vi "Get Channels From Line.vi"(11 "Line":T1) -> (2 "Channels":refnum<class "TBM channel.lvclass">[](array[class]), 3 "Line 2":T1)   [LabVIEW 2013, in "Modbus Module configuration.lvclass"]
uses:
  Modbus Module configuration.lvclass
  module channel/Modbus Module Channel.lvclass
  Line.ctl
  <vilib>/NI/Tag Bus Module Framework/channel/TBM channel.lvclass
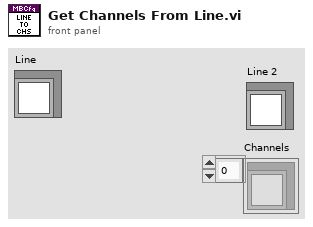
[diagram p1: front panel]
types:
  T1 = typedef "Modbus Module configuration.lvclass/Line.ctl" = refnum<class "Modbus Module Channel.lvclass">
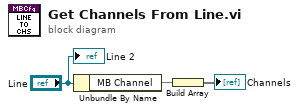
[diagram p0: block diagram]
diagram:
  n1 = Unbundle By Name("Line") -> ("MB Channel"=w3)
  n2 = Build Array(w3) -> (→"Channels":void[])
  "Line 2" <- "Line"
